vi "SettingsPanel.vi"(8 "error in":errorcluster, 11 "Settings In":T2={"Harware Configuration"={"Camera"="cam1", "Frames Per Second"=15, "Simulate Recording"=FALSE, "Simulated Recording Sample"=path "", "Timestamp Method"=enum."Camera Timestamp"}, "Base Recording Path"=path "", "Type Of Recording"="", "Recording Codec"="", "TrackingSettings"={"Max Radius"=10, "Threshold"=160.0, "ROI"={"Left"=0, "Top"=0, "Right"=0, "Bottom"=0, "Rotation"=0.0}}, "Calibration"={"Pixel Width (X)"=1.0, "Pixel Height (Y)"=1.0}, "Broadcast Length"=0} {"Broadcast Length" min=0; "TrackingSettings"."ROI"."Rotation" format="%.2f"; "TrackingSettings"."ROI"."Left" scale=0.0..1024.0; "TrackingSettings"."ROI"."Right" scale=0.0..1024.0; "TrackingSettings"."Threshold" scale=0.0..255.0}) -> (0 "error out":errorcluster, 2 "Canceled?":bool, 3 "Settings Out":T2={"Harware Configuration"={"Camera"="cam1", "Frames Per Second"=15, "Simulate Recording"=FALSE, "Simulated Recording Sample"=path "", "Timestamp Method"=enum."Camera Timestamp"}, "Base Recording Path"=path "", "Type Of Recording"="", "Recording Codec"="", "TrackingSettings"={"Max Radius"=0, "Threshold"=160.0, "ROI"={"Left"=0, "Top"=0, "Right"=0, "Bottom"=0, "Rotation"=0.0}}, "Calibration"={"Pixel Width (X)"=1.0, "Pixel Height (Y)"=1.0}, "Broadcast Length"=0} {"Broadcast Length" min=0; "TrackingSettings"."ROI"."Rotation" format="%.2f"; "TrackingSettings"."ROI"."Left" scale=0.0..1024.0; "TrackingSettings"."ROI"."Right" scale=0.0..1024.0; "TrackingSettings"."Threshold" scale=0.0..255.0})   [LabVIEW 2017, in "ImageAcquisitionLibrary.lvlib"]
uses:
  ImageAcquisitionLibrary.lvlib
  <vilib>/userdefined/High Color/IMAQdx.ctl
  Settings.ctl
  Tracking/TrackingSettings.ctl
  Calibration.ctl
  <vilib>/vision/Image Controls.llb/IMAQ Image.ctl
panel:
  in  "Calibration":T1={"Pixel Width (X)"=1.0, "Pixel Height (Y)"=1.0} {"Pixel Width (X)" format="%.0p"; "Pixel Height (Y)" format="%.0p"}
  in  "Tracking Settings":bool
  in  "Type Of Recording":string(combo)="Snapshot"
  in  "fps":dbl=15.0
  in  "Camera":T3
  in  "Simulate":bool
  in  "Simulated Acquisition Sample":path=path "D:/Dropbox/Colloids/2015-06-15/ImageAcquisitionProgram/SimulationInput/SampleImage.jpg"
  in  "Recording Path":path=path "C:/Users/aortiza/Desktop"
  in  "Codex":string(combo)="Y800 Uncompressed Grey Scale (NI Vision)"
  in  "Cancel Button":bool
  in  "OK Button":bool
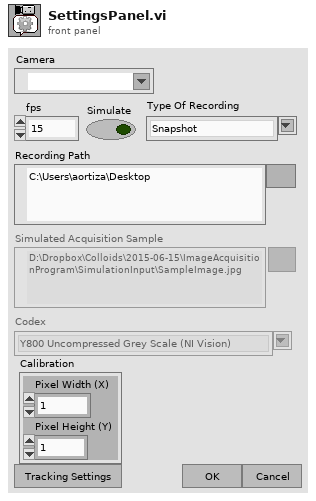
[diagram p1: front panel]
types:
  T1 = typedef "ImageAcquisitionLibrary.lvlib/Calibration.ctl" = cluster{"Pixel Width (X)":dbl, "Pixel Height (Y)":dbl}
  T2 = typedef "ImageAcquisitionLibrary.lvlib/Settings.ctl" = cluster{"Harware Configuration":cluster{"Camera":T3, "Frames Per Second":u32, "Simulate Recording":bool, "Simulated Recording Sample":path, "Timestamp Method":enum16{"System Timestamp", "Camera Timestamp", "IMAQdx Timestamp"}}, "Base Recording Path":path, "Type Of Recording":string, "Recording Codec":string, "TrackingSettings":T4, "Calibration":T1, "Broadcast Length":i32}
  T3 = typedef "IMAQdx.ctl" = refnum<k21>
  T4 = typedef "ImageAcquisitionLibrary.lvlib/TrackingSettings.ctl" = cluster{"Max Radius":i32, "Threshold":sgl, "ROI":T5}
  T5 = typedef "IMAQ Rectangle" = cluster{"Left":i32, "Top":i32, "Right":i32, "Bottom":i32, "Rotation":dbl}
  T6 = typedef "IMAQ Image.ctl" = refnum<image>
  T7 = enum8{"Enabled", "Disabled", "Disabled and Grayed Out"}
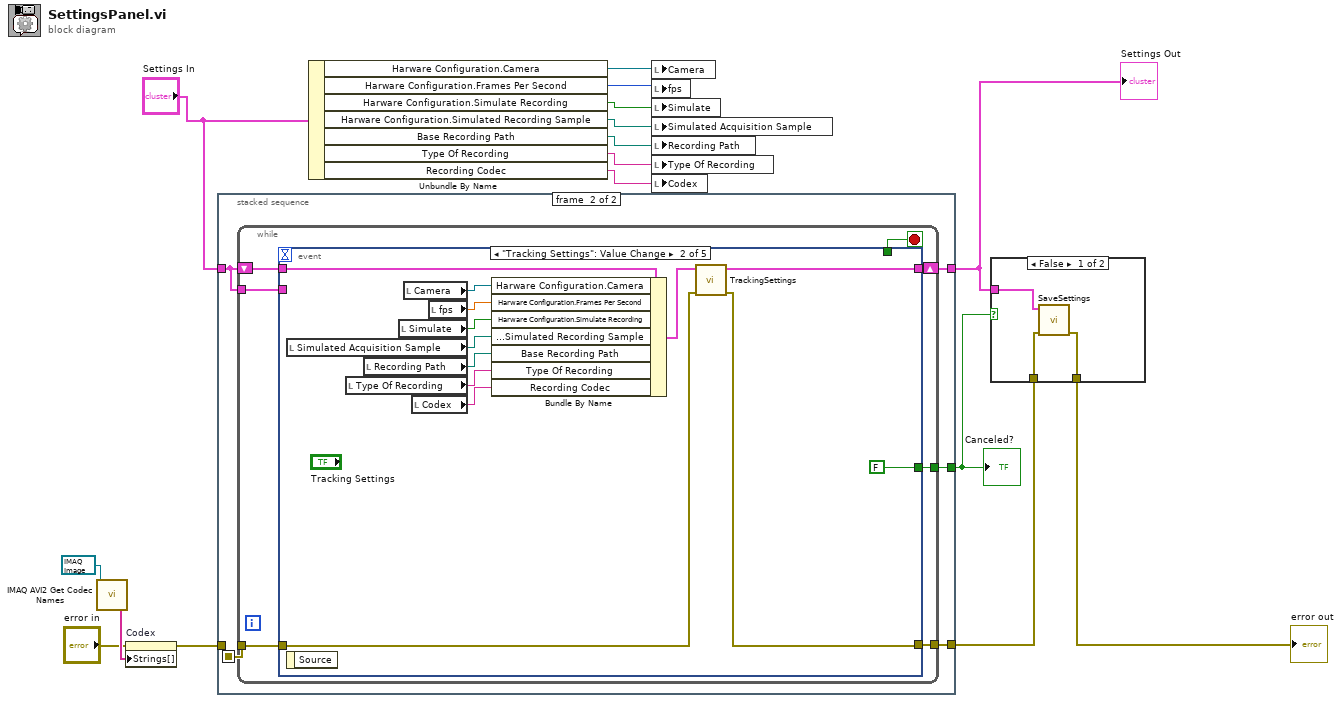
[diagram p0: block diagram]
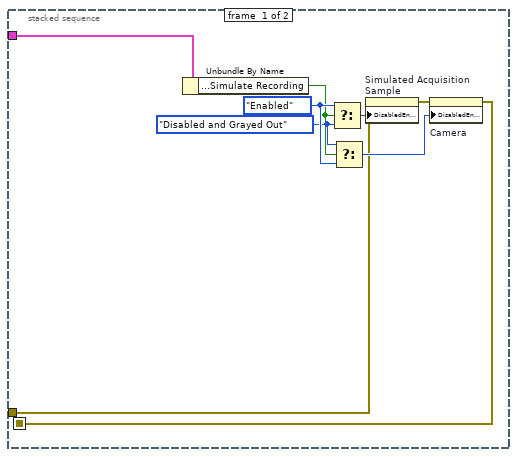
[diagram p2: hidden frame]
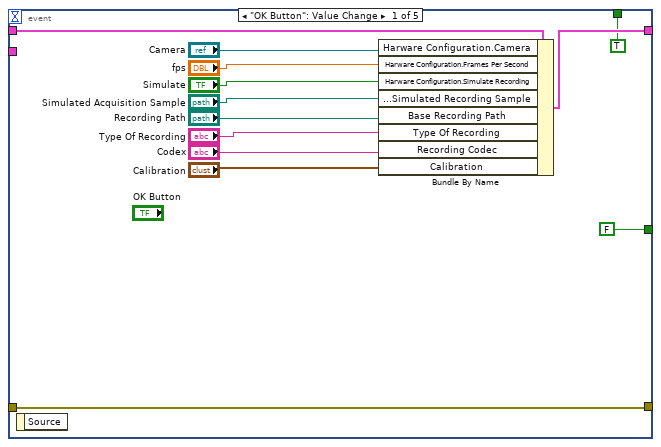
[diagram p3: hidden frame]
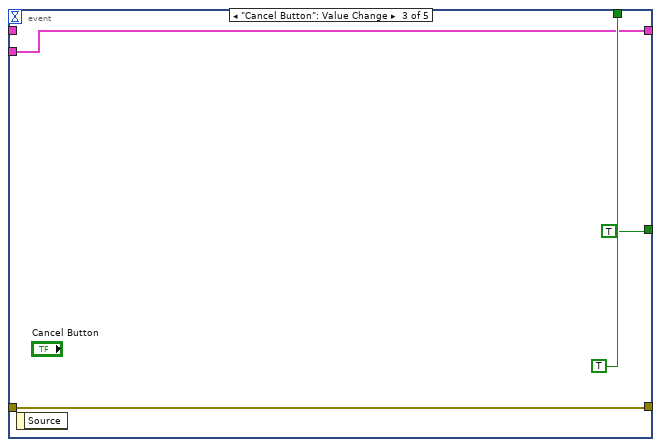
[diagram p4: hidden frame]
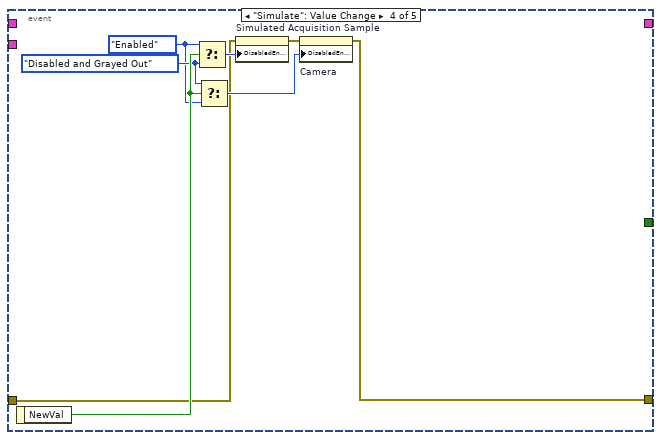
[diagram p5: hidden frame]
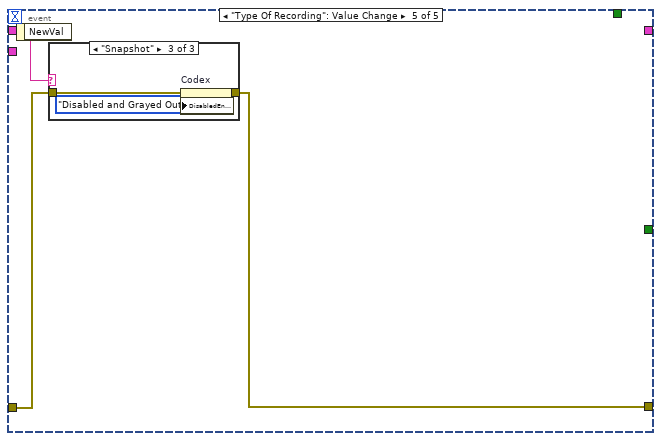
[diagram p6: hidden frame]
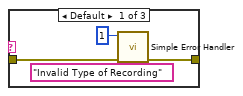
[diagram p7: hidden frame]
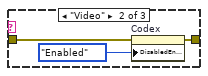
[diagram p8: hidden frame]
diagram:
  n1 = call "IMAQ AVI2 Get Codec Names"("Image"=T6 refnum) -> ("Codec Names"=w7:string[])  [unwired: 9 in, 1 out]
  n2 = property on="Codex" class="CmbBox"(error in="error in", "Strings[]"=w7) -> (error out=w5:errorcluster)  [unwired: 1 in, 1 out]
  n3 = stacked-sequence {
    seq-local: [w17 _] -> [_ w27]
    tunnel: "Settings In" -> [w21 w26]
    tunnel: w5 -> [w18 _]
    tunnel: [_ w30] -> w1
    tunnel: [_ w29] -> w4
    tunnel: [_ w28] -> w3
    frame #0 {
      w19 = T7."Disabled and Grayed Out" ("Disabled")
      w22 = T7."Enabled" ("Disabled")
      n4 = Unbundle By Name(w21) -> ("Harware Configuration.Simulate Recording"=w20:bool)
      n5 = Select(t=w22, s=w20, f=w19) -> (s? t:f=w25:T7)
      n6 = Select(t=w19, s=w20, f=w22) -> (s? t:f=w24:T7)
      n7 = property on="Simulated Acquisition Sample" class="Path"(error in=w18, "DisabledEnum"=w25) -> (error out=w23:errorcluster)  [unwired: 1 in, 1 out]
      n8 = property on="Camera" class="IMAQdx (strict)"(error in=w23, "DisabledEnum"=w24) -> (error out=w17:errorcluster)  [unwired: 1 in, 1 out]
    }
    frame #1 {
      n9 = while {
        shift-right: [w31] -> w29
        shift-left: w26 -> [w37]
        tunnel: [w35] -> w30
        tunnel: [w34] -> w28
        tunnel: w27 -> [w33]
        tunnel: w26 -> [w32]
        stop <- w36 stop-if-true
        n10 = event shown="[1] \"Tracking Settings\": Value Change" {
          selector: _ -> [_ _ _ _ _]
          dyn-events: _ -> [_ _ _ _ _]
          timeout: _ -> [_ _ _ _ _]
          tunnel: w37 -> [w50 w63 _ _ _]
          tunnel: [TRUE _ TRUE _ _] -> w36
          tunnel: [FALSE FALSE TRUE _ _] -> w35
          tunnel: [w38 w58 w65 w71 w77] -> w34
          tunnel: w33 -> [w38 w59 w65 w68 w76]
          tunnel: w32 -> [_ _ w64 _ _]
          tunnel: [w45 w60 w64 _ _] -> w31
          event "OK Button": Value Change {
            n11 = event-data() -> ()  [unwired: 1 in, 1 out]
            n12 = Bundle By Name(cluster=w50, "Harware Configuration.Camera"="Camera", "Harware Configuration.Frames Per Second"="fps", "Harware Configuration.Simulate Recording"="Simulate", "Harware Configuration.Simulated Recording Sample"="Simulated Acquisition Sample", "Base Recording Path"="Recording Path", "Type Of Recording"="Type Of Recording", "Recording Codec"="Codex", "Calibration"="Calibration") -> (w45:T2)
          }
          event "Tracking Settings": Value Change {
            n13 = local read "Simulated Acquisition Sample"() -> (w54:path)
            n14 = event-data() -> ()  [unwired: 1 in, 1 out]
            n15 = local read "Type Of Recording"() -> (w56:string)
            n16 = local read "Recording Path"() -> (w55:path)
            n17 = local read "Simulate"() -> (w53:bool)
            n18 = local read "Camera"() -> (w51:T3)
            n19 = local read "Codex"() -> (w57:string)
            n20 = local read "fps"() -> (w52:dbl)
            n21 = Bundle By Name(cluster=w63, "Harware Configuration.Camera"=w51, "Harware Configuration.Frames Per Second"=w52, "Harware Configuration.Simulate Recording"=w53, "Harware Configuration.Simulated Recording Sample"=w54, "Base Recording Path"=w55, "Type Of Recording"=w56, "Recording Codec"=w57) -> (w61:T2)
            n22 = call "TrackingSettings.vi"("error in"=w59, "Settings In"=w61) -> ("error out"=w58:errorcluster, "Settings Out"=w60:T2)  [unwired: 7 in, 1 out]
          }
          event "Cancel Button": Value Change {
            n23 = event-data() -> ()  [unwired: 1 in, 1 out]
          }
          event "Simulate": Value Change {
            w70 = T7."Disabled and Grayed Out" ("Disabled")
            w69 = T7."Enabled" ("Disabled")
            n24 = event-data() -> ("NewVal"=w74:bool)  [unwired: 1 in]
            n25 = Select(t=w69, s=w74, f=w70) -> (s? t:f=w75:T7)
            n26 = Select(t=w70, s=w74, f=w69) -> (s? t:f=w73:T7)
            n27 = property on="Simulated Acquisition Sample" class="Path"(error in=w68, "DisabledEnum"=w75) -> (error out=w72:errorcluster)  [unwired: 1 in, 1 out]
            n28 = property on="Camera" class="IMAQdx (strict)"(error in=w72, "DisabledEnum"=w73) -> (error out=w71:errorcluster)  [unwired: 1 in, 1 out]
          }
          event "Type Of Recording": Value Change {
            n29 = event-data() -> ("NewVal"=w78:string)  [unwired: 1 in]
            n30 = case shown="\"Snapshot\"" w78 {
              tunnel: [w81 w83 w87] -> w77
              tunnel: w76 -> [w82 w84 w86]
              frame Default {
                n31 = call <vilib>:"Simple Error Handler.vi"("error code (no error:0)"=1, "error source (\" \")"="Invalid Type of Recording" ("error source (\" \")"), "error in (no error)"=w82) -> ("error out"=w81:errorcluster)  [unwired: 2 in, 4 out]
              }
              frame "Video" {
                n32 = property on="Codex" class="CmbBox"(error in=w84, "DisabledEnum"=T7."Enabled" ("Disabled")) -> (error out=w83:errorcluster)  [unwired: 1 in, 1 out]
              }
              frame "Snapshot" {
                n33 = property on="Codex" class="CmbBox"(error in=w86, "DisabledEnum"=T7."Disabled and Grayed Out" ("Disabled")) -> (error out=w87:errorcluster)  [unwired: 1 in, 1 out]
              }
            }
          }
        }
      }
    }
  }
  "Settings Out" <- w4
  "Canceled?" <- w1
  n34 = Unbundle By Name("Settings In") -> ("Harware Configuration.Camera"=w14:T3, "Harware Configuration.Frames Per Second"=w13:u32, "Harware Configuration.Simulate Recording"=w12:bool, "Harware Configuration.Simulated Recording Sample"=w10:path, "Base Recording Path"=w11:path, "Type Of Recording"=w9:string, "Recording Codec"=w8:string)
  n35 = local write "Camera"(w14) -> ()
  n36 = local write "fps"(w13) -> ()
  n37 = local write "Simulate"(w12) -> ()
  n38 = local write "Simulated Acquisition Sample"(w10) -> ()
  n39 = local write "Recording Path"(w11) -> ()
  n40 = local write "Type Of Recording"(w9) -> ()
  n41 = local write "Codex"(w8) -> ()
  n42 = case shown="False" w1 {
    tunnel: w4 -> [w91 _]
    tunnel: w3 -> [w90 w92]
    tunnel: [w89 w92] -> w2
    frame False {
      n43 = call "SaveSettings.vi"("error in (no error)"=w90, "Settings"=w91) -> ("error out"=w89:errorcluster)  [unwired: 9 in]
    }
    frame True {
    }
  }
  "error out" <- w2
